vi "Ball_possession.vi"(10 "balls":T1[](array[typedef]), 11 "IA State":T2={"our_robots"=[], "enemy_robots"=[], "balls"=[], "geometry"={"field_length"=0, "field_width"=0, "goal_width"=0, "goal_depth"=0, "center_circle_radius"=0, "defense_width"=0, "defense_depth"=0, "free_kick_from_defense_dist"=0, "penalty_spot_from_field_line_dist"=0, "penalty_line_from_spot_dist"=0, "half_moon_depth"=0, "half_moon_width"=0}, "IA Judge"={"stage"="", "command"="", "our_goalie_id"=0.0, "enemy_goalie_id"=0.0, "command enum"=enum."Halt", "Time"=enum."Azul"}, "Received Timestamp"=timestamp(0 s since 1904-01-01), "Events"={"Touch"=FALSE, "id touch"=0.0, "Ball out of \nVision"=FALSE, "Ball inside \nGoalie area"=FALSE, "Robot not responding"=FALSE, "Robots responding status"=[1.0, 1.0, 1.0, 1.0, 1.0, 1.0], "Enemy Ball \nPossession"=FALSE, "Id ini Possession"=0.0, "Ball Possesion"=FALSE, "Id Possesion"=0.0, "Ball at\nour goal side"=FALSE, "Ball at\ntouchline"=FALSE, "Ball at\nenemy goal side"=FALSE}}) -> (2 "id":u32, 3 "Boolean":bool)   [LabVIEW 2018]
uses:
  Core/AI Input.ctl
  Core/AI Robot.ctl
  Functions Enum.ctl
  AttackerStates.ctl
  Path Planning/RRT/PathDests.ctl
  Path Planning/RRT/PathDest.ctl
  Core/AI Ball.ctl
  Core/Field Size.ctl
  Core/AI Judge.ctl
  Command Enum.ctl
  Util/Events/Events.ctl
  <vilib>/Analysis/coordinate.llb/Wrap Angle (scalar).vi
  <vilib>/Analysis/_algsub.llb/Real Vector Norm.vi
  <vilib>/Analysis/NI_AALPro.lvlib
  <vilib>/Analysis/NI_AAL_Angle.lvlib
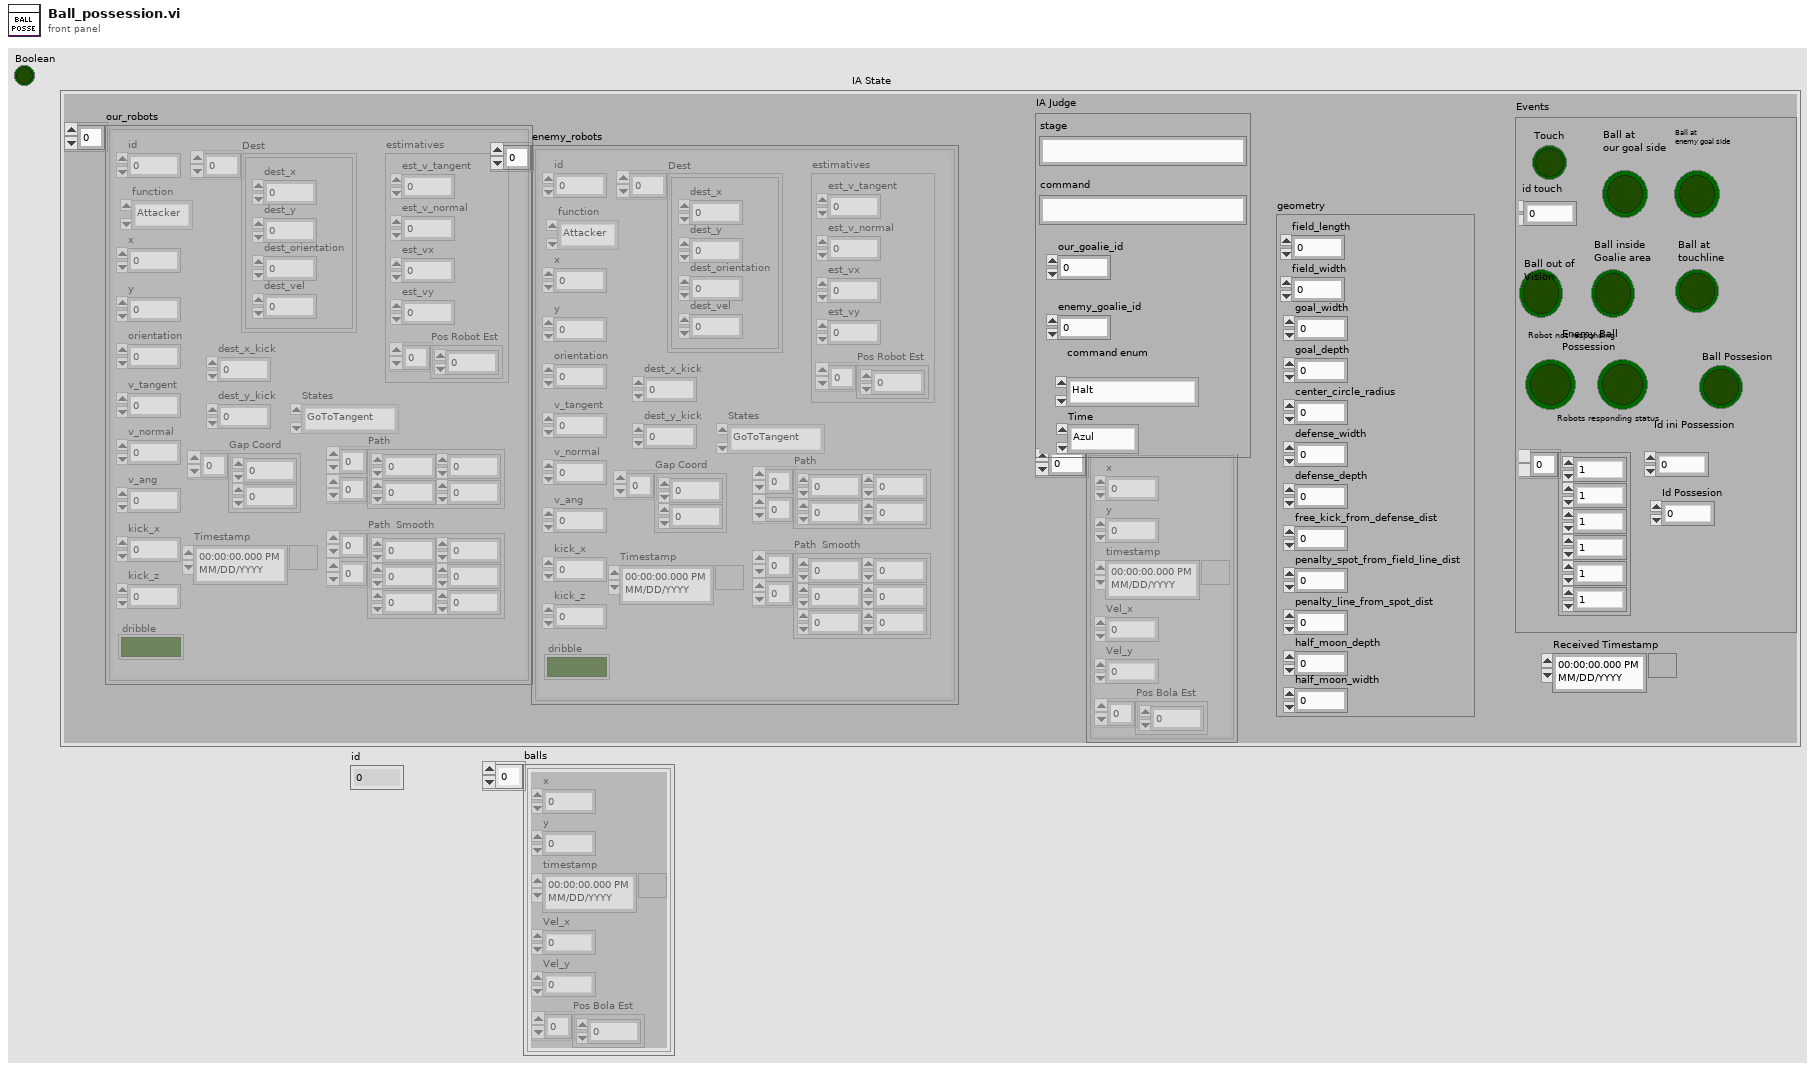
[diagram p1: front panel]
types:
  T1 = typedef "AI Ball.ctl" = cluster{"x":dbl, "y":dbl, "timestamp":timestamp, "Vel_x":dbl, "Vel_y":dbl, "Pos Bola Est":dbl[]}
  T2 = typedef "AI Input.ctl" = cluster{"our_robots":T3[], "enemy_robots":T3[], "balls":T1[], "geometry":T8, "IA Judge":T9, "Received Timestamp":timestamp, "Events":T11}
  T3 = typedef "AI Robot.ctl" = cluster{"id":u32, "function":T4, "x":dbl, "y":dbl, "orientation":dbl, "v_tangent":dbl, "v_normal":dbl, "v_ang":dbl, "kick_x":dbl, "kick_z":dbl, "dribble":bool, "Timestamp":timestamp, "estimatives":cluster{"est_v_tangent":dbl, "est_v_normal":dbl, "est_vx":dbl, "est_vy":dbl, "Pos Robot Est":dbl[]}, "dest_x_kick":dbl, "dest_y_kick":dbl, "Gap Coord":dbl[], "States":T5, "Path ":dbl[][], "Path  Smooth":dbl[][], "Dest":T6}
  T4 = typedef "Functions Enum.ctl" = enum16{"Attacker", "Goalie", "Defender", "Striker", "Goto 0", "Dummy", "Kicker", "ZigZag"}
  T5 = typedef "AttackerStates.ctl" = enum16{"Pass", "GoToTangent", "BallGetting", "GoToKick", "Rotate anti-clockwise", "Rotate Clockwise", ""}
  T6 = typedef "PathDests.ctl" = T7[]
  T7 = typedef "PathDest.ctl" = cluster{"dest_x":dbl, "dest_y":dbl, "dest_orientation":dbl, "dest_vel":dbl}
  T8 = typedef "Field Size.ctl" = cluster{"field_length":u32, "field_width":u32, "goal_width":u32, "goal_depth":u32, "center_circle_radius":u32, "defense_width":u32, "defense_depth":u32, "free_kick_from_defense_dist":u32, "penalty_spot_from_field_line_dist":u32, "penalty_line_from_spot_dist":u32, "half_moon_depth":u32, "half_moon_width":u32}
  T9 = typedef "AI Judge.ctl" = cluster{"stage":string, "command":string, "our_goalie_id":dbl, "enemy_goalie_id":dbl, "command enum":T10, "Time":enum16{"Azul", "Amarelo"}}
  T10 = typedef "Command Enum.ctl" = enum16{"Halt", "Stop", "Force Start", "PKA Normal Start", "Prepare Kickoff Ally", "PKE Normal Start", "Prepare Kickoff Enemy", "Prepare Penalty Ally", "PPA Normal Start", "Prepare Penalty Enemy", "PPE Normal Start", "Ball Placement Enemy Up", "Ball Placement Enemy Down", "Ball Placement Ally Up", "Ball Placement Ally Mid", "Ball Placement Ally Down", "Indirect Free Enemy", "Indirect Free Ally", "Timeout Enemy", "Timeout Ally", "Goal Enemy", "Goal Ally", "Normal Half Time", "Extra Time Break", "Extra Half Time", "None", "Post Game"}
  T11 = typedef "Events.ctl" = cluster{"Touch":bool, "id touch":dbl, "Ball out of \nVision":bool, "Ball inside \nGoalie area":bool, "Robot not responding":bool, "Robots responding status":dbl[], "Enemy Ball \nPossession":bool, "Id ini Possession":dbl, "Ball Possesion":bool, "Id Possesion":dbl, "Ball at\nour goal side":bool, "Ball at\ntouchline":bool, "Ball at\nenemy goal side":bool}
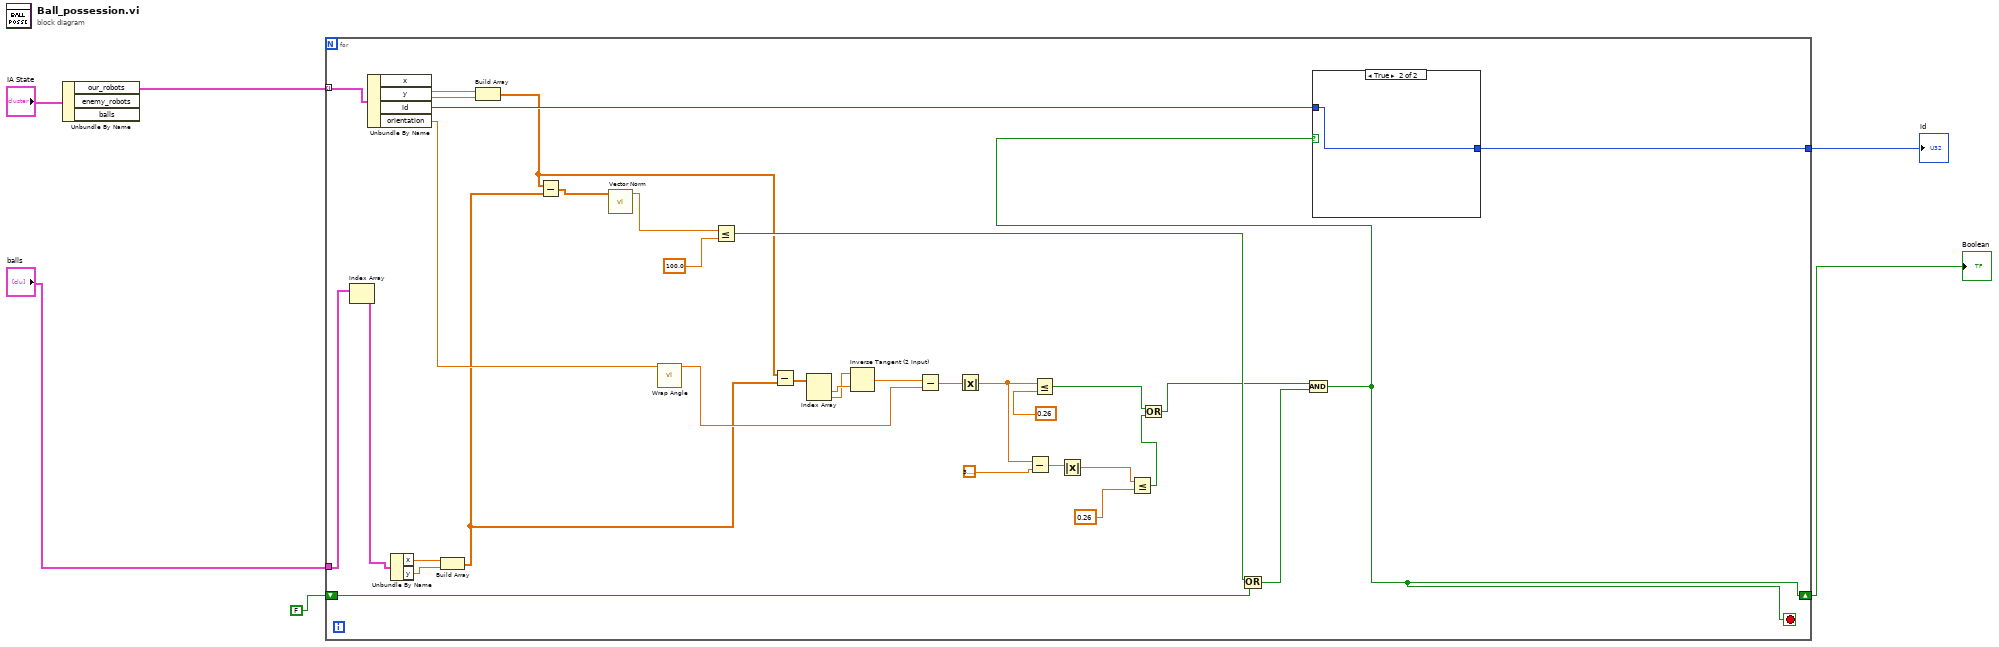
[diagram p0: block diagram]
diagram:
  n1 = Unbundle By Name("IA State") -> ("our_robots"=w5:T3[])  [unwired: 2 out]
  n2 = for {
    tunnel: w5 -> [w40] mode=indexing
    tunnel: "balls" -> [w31]
    shift-right: [w15] -> w2
    shift-left: FALSE -> [w32]
    tunnel: [w27] -> w1
    stop <- w15 stop-if-true
    n3 = Index Array(array=w31) -> (element=w30:T1)  [unwired: 1 in]
    n4 = Unbundle By Name(w40) -> ("x"=w39:dbl, "y"=w38:dbl, "id"=w28:u32, "orientation"=w20:dbl)
    n5 = Unbundle By Name(w30) -> ("x"=w37:dbl, "y"=w36:dbl)
    n6 = Build Array(w37, w36) -> (w19:dbl[])
    n7 = Build Array(w39, w38) -> (w21:dbl[])
    n8 = Subtract(x=w21, y=w19) -> (x-y=w35:dbl[])
    n9 = call-poly <vilib>:"Vector Norm.vi"("Input Vector"=w35) -> ("norm"=w34:dbl)  [unwired: 9 in, 1 out]
    n10 = call-poly <vilib>:"Wrap Angle.vi"("angle in"=w20) -> ("angle out"=w22:dbl)  [unwired: 9 in, 1 out]
    n11 = Less Or Equal?(x=w34, y=100.0) -> (x <= y?=w29:bool)
    n12 = Subtract(x=w21, y=w19) -> (x-y=w24:dbl[])
    n13 = Index Array(array=w24) -> (element #1=w26:dbl, element #2=w25:dbl)  [unwired: 2 in]
    n14 = Inverse Tangent (2 Input)(1:w26, 2:w25) -> (0:w23:dbl)
    n15 = Subtract(x=w23, y=w22) -> (x-y=w18:dbl)
    n16 = Absolute Value(x=w18) -> (abs(x)=w14:dbl)
    n17 = Subtract(x=w14, y=3.141592653589793) -> (x-y=w12:dbl)
    n18 = Less Or Equal?(x=w14, y=0.26) -> (x <= y?=w9:bool)
    n19 = Absolute Value(x=w12) -> (abs(x)=w11:dbl)
    n20 = Less Or Equal?(x=w11, y=0.26) -> (x <= y?=w8:bool)
    n21 = Or(x=w9, y=w8) -> (x .or. y?=w7:bool)
    n22 = Or(x=w29, y=w32) -> (x .or. y?=w16:bool)
    n23 = And(x=w7, y=w16) -> (x .and. y?=w15:bool)
    n24 = case shown="True" w15 {
      tunnel: w28 -> [_ w41]
      tunnel: [_ w41] -> w27
      frame False {
      }
      frame True {
      }
    }
  }
  "Boolean" <- w2
  "id" <- w1
